vi "Closing Sequence For Review.vi"(8 "error in (no error)":errorcluster, 10 "tdms file":refnum<k34>, 11 "Notifier in":refnum<notifier>) -> ()   [LabVIEW 2020]
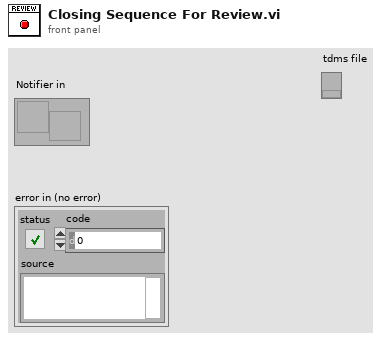
[diagram p1: front panel]
types:
  T1 = cluster{"notification":string, "Variant":variant}
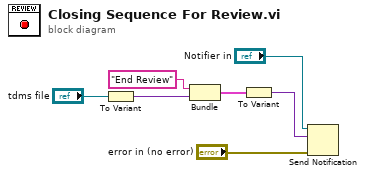
[diagram p0: block diagram]
diagram:
  n1 = To Variant(anything="tdms file") -> (Variant=w1:variant)
  n2 = Bundle("notification"="End Review", "Variant"=w1) -> (w4:T1)  [unwired: 1 in]
  n3 = To Variant(anything=w4) -> (Variant=w3:variant)
  n4 = Send Notification(notification=w3, notifier="Notifier in", error in (no error)="error in (no error)") -> ()  [unwired: 2 out]
